vi "Configure OAuth.vi"(5 "Oauth2 in":refnum<class "Oauth2.lvclass">, 7 "Grant Flow":T1, 8 "scopes":string[](array[string]), 9 "Client Secret":string, 10 "Client ID":string, 11 "Authorization Server URI":string) -> (0 "error out":errorcluster, 3 "Oauth2":refnum<class "Oauth2.lvclass">)   [LabVIEW 2013, in "Oauth2.lvclass"]
uses:
  Oauth2.lvclass
  OAuth2 Flow -- enum.ctl
  <vilib>/LabVIEW Open Source Project/OpenURI/uri/URI.lvclass
  OAuthToken/OAuth2 Token Element -- enum.ctl
  Oauth2.lvclass/Oauth2.ctl
  <vilib>/LabVIEW Open Source Project/OpenURI/uri/Get URI.vi
  OAuthToken/OAuthAccessToken.lvclass
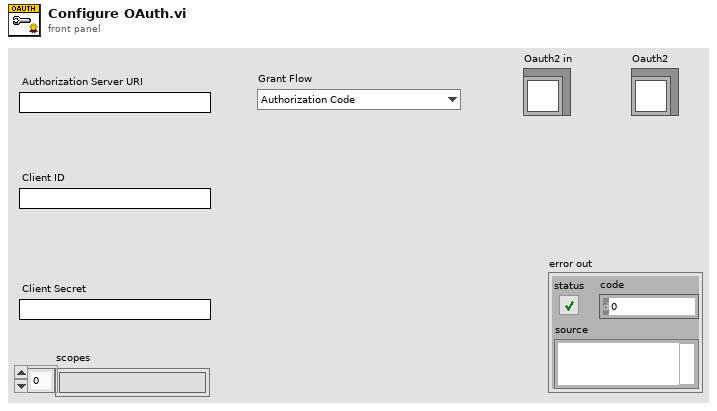
[diagram p1: front panel]
types:
  T1 = typedef "Oauth2.lvclass/OAuth2 Flow -- enum.ctl" = enum16{"Authorization Code", "Authorization Code (PKCE)", "Implicit", "Resource Owner Credentials", "Client Credentials"}
  T2 = typedef "OAuthAccessToken.lvclass/OAuth2 Token Element -- enum.ctl" = enum16{"client_id", "client_secret", "response_type", "scope", "redirect_uri", "error", "error_description", "error_uri", "grant_type", "code", "access_token", "token_type", "expires_in", "username", "password", "refresh_token", "endpoint element"}
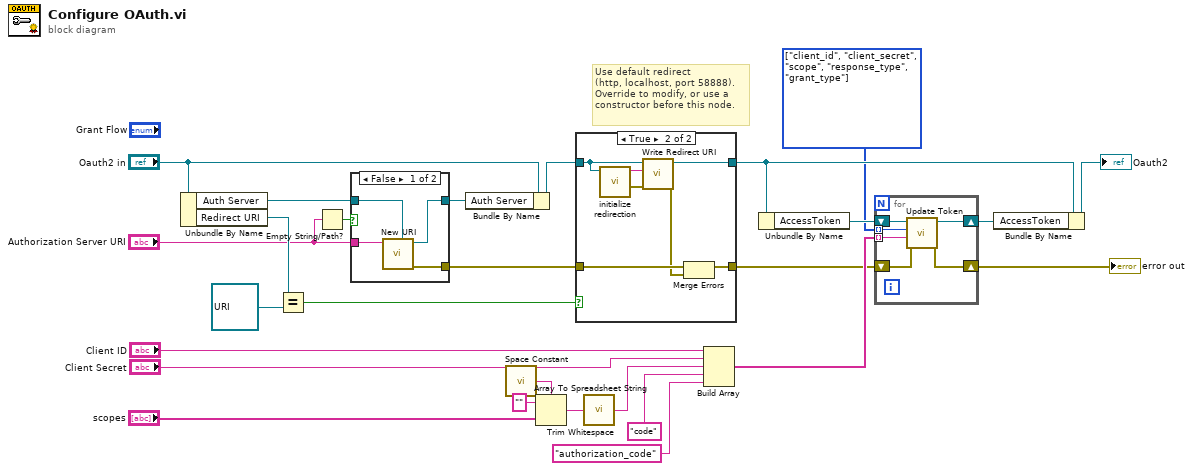
[diagram p0: block diagram]
diagram:
  w10 = T2[] [enum."client_id", enum."client_secret", enum."scope", enum."response_type", enum."grant_type"] items=["client_id", "client_secret", "response_type", "scope", "redirect_uri", "error", "error_description", "error_uri", "grant_type", "code", "access_token", "token_type", "expires_in", "username", "password", "refresh_token", "endpoint element"]
  # "Use default redirect\n(http, localhost, port 58888).\nOverride to modify, or use a\nconstructor before this node."
  n1 = Unbundle By Name("Oauth2 in") -> ("Auth Server"=w24:refnum<class "URI.lvclass">, "Redirect URI"=w25:refnum<class "URI.lvclass">)
  n2 = Equal?(x=w25, y=refnum<class "URI.lvclass"> refnum ("x")) -> (x = y?=w26:bool)
  n3 = Empty String/Path?(string/path="Authorization Server URI") -> (empty?=w19:bool)
  n4 = case shown="False" w19 {
    tunnel: w24 -> [w31 w32]
    tunnel: [w30 w32] -> w23
    tunnel: "Authorization Server URI" -> [w29 _]
    tunnel: [w28 _] -> w4
    frame False {
      n5 = call <vilib>:"New URI.vi"("URI in"=w31, "URI"=w29) -> ("error out"=w28:errorcluster, "URI"=w30:refnum<class "URI.lvclass">)  [unwired: 8 in]
    }
    frame True {
    }
  }
  n6 = Bundle By Name(cluster="Oauth2 in", "Auth Server"=w23) -> (w21:refnum<class "Oauth2.lvclass">)
  n7 = call <vilib>:"Space Constant.vi"() -> ("String"=w14:string)
  n8 = Array To Spreadsheet String(delimiter (Tab)=w14, array="scopes", 3:"" ("format string")) -> (spreadsheet string=w15:string)
  n9 = case shown="True" w26 {
    tunnel: w21 -> [w34 w38]
    tunnel: [w34 w41] -> w17
    tunnel: [w33 w36] -> w3
    tunnel: w4 -> [w33 w37]
    frame False {
    }
    frame True {
      n10 = call-dynamic "initialize redirection.vi"("Oauth2"=w38) -> ("error out"=w39:errorcluster, "Redirect URI"=w40:string)  [unwired: 9 in]
      n11 = call "Write Redirect URI.vi"("error in (no error)"=w39, "Redirect URI"=w40, "Oauth2 in"=w38) -> ("error out"=w35:errorcluster, "Oauth2 out"=w41:refnum<class "Oauth2.lvclass">)  [unwired: 7 in]
      n12 = Merge Errors(w37, w35) -> (w36:errorcluster)
    }
  }
  n13 = call <vilib>:"Trim Whitespace.vi"("string"=w15) -> ("trimmed string"=w6:string)  [unwired: 1 in]
  n14 = Build Array("Client ID", "Client Secret", w6, "code" ("argument"), "authorization_code" ("argument")) -> (w7:string[])
  n15 = Unbundle By Name(w17) -> ("AccessToken"=w18:refnum<class "OAuthAccessToken.lvclass">)
  n16 = for {
    tunnel: w7 -> [w46] mode=indexing
    shift-right: [w45] -> w11
    shift-left: w18 -> [w47]
    tunnel: w10 -> [w44] mode=indexing
    shift-right: [w42] -> w2
    shift-left: w3 -> [w43]
    n17 = call "Update Token.vi"("error in (no error)"=w43, "Value"=w46, "Token element"=w44, "OAuthAccessToken in"=w47) -> ("error out"=w42:errorcluster, "OAuthAccessToken out"=w45:refnum<class "OAuthAccessToken.lvclass">)  [unwired: 6 in]
  }
  "error out" <- w2
  n18 = Bundle By Name(cluster=w17, "AccessToken"=w11) -> (→"Oauth2":refnum<class "Oauth2.lvclass">)
